vi "New.vi"(4 "Plugin":refnum<class "Plugin.lvclass">, 5 "FIFO Options":T1, 6 "Logging Interface":refnum<class "Logging Interface.lvclass">, 7 "thread ID":u8, 8 "error in (no error)":errorcluster, 10 "Thread Configuration":refnum<class "Thread Configuration.lvclass">, 11 "Plugin Thread type":refnum<class "Plugin Thread.lvclass">) -> (0 "error out":errorcluster, 2 "Plugin Thread Interface":refnum<class "Plugin Interface.lvclass">, 3 "Plugin Thread out":refnum<class "Plugin Thread.lvclass">)   [LabVIEW 2019, in "DSF Core.lvlib" / "Plugin Thread.lvclass"]
uses:
  Thread/Plugin/Plugin Thread.lvclass
  C:/Dev/GitHub/niveristand-data-sharing-framework-custom-device/Core/Classes/Thread/Thread.lvclass
  Interface/Plugin/Plugin Interface.lvclass
  C:/Dev/GitHub/niveristand-data-sharing-framework-custom-device/Core/Classes/Interface/Interface.lvclass
  Configuration/Core/Thread/Thread Configuration.lvclass
  Interface/Logging/Logging Interface.lvclass
  Plugin/Plugin.lvclass
  Typedefs/DSF FIFO Options.ctl
  Interface/Interface.lvclass/Interface.ctl
  Thread/Thread.lvclass/Thread.ctl
  Plugin/Plugin.lvclass/Plugin.ctl
  Timing/Timing.lvclass/Timing.ctl
  Thread/Thread Settings.ctl
  Thread/Plugin/Plugin Thread.lvclass/Plugin Thread.ctl
  Interface/New Interface.vi
  Interface/Create RT FIFO.vi
  Thread/Thread.lvclass
  Timing/Timing.lvclass
  Framework/Framework.lvclass
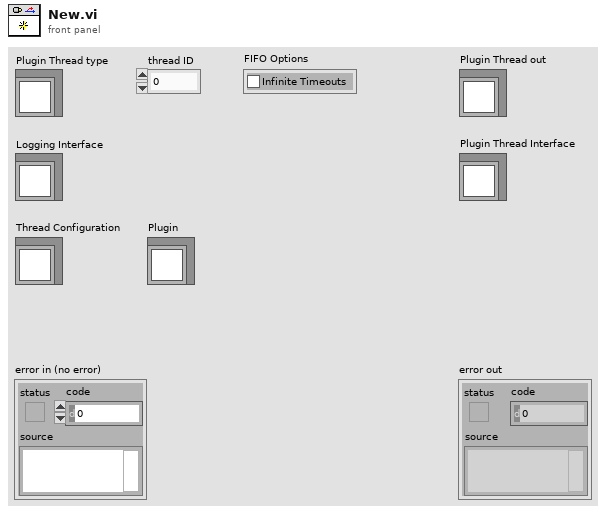
[diagram p1: front panel]
types:
  T1 = typedef "DSF Core.lvlib/Framework.lvclass/DSF FIFO Options.ctl" = cluster{"Infinite Timeouts":bool}
  T2 = typedef "DSF Core.lvlib/Thread.lvclass/Thread Settings.ctl" = cluster{"Priority":u16, "Processor":i32}
  T3 = typedef "DSF Core.lvlib/Thread Configuration.lvclass/Core Thread Configuration.ctl" = cluster{"processor":i32, "priority offset":i16}
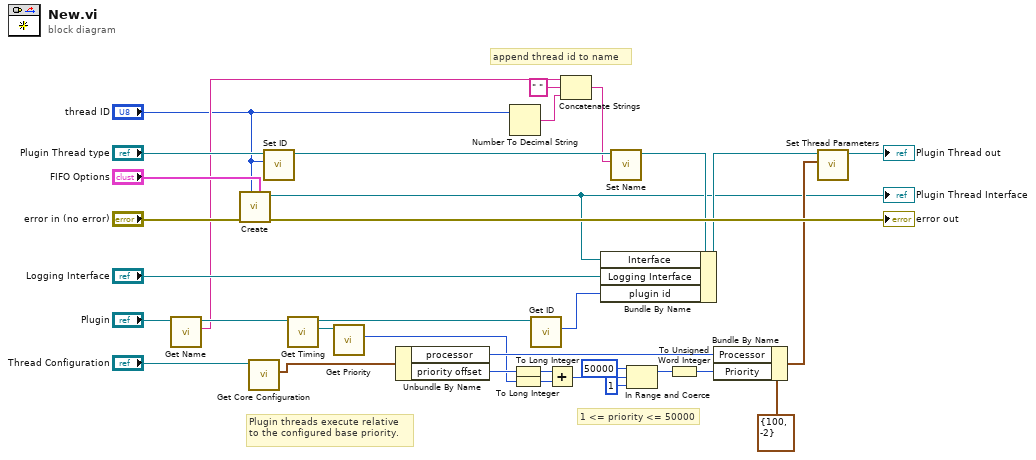
[diagram p0: block diagram]
diagram:
  # "1 <= priority <= 50000"
  # "append thread id to name"
  # "Plugin threads execute relative to the configured base priority."
  n1 = call "Get Name.vi"("Plugin in"="Plugin") -> ("name"=w4:string, "Plugin out"=w12:refnum<class "Plugin.lvclass">)  [unwired: 9 in]
  n2 = call "Create.vi"("fifo options"="FIFO Options", "id (0)"="thread ID", "error in (no error)"="error in (no error)") -> ("error out"=→"error out":errorcluster, "Plugin Interface"=w6:refnum<class "Plugin Interface.lvclass">)  [unwired: 7 in]
  "Plugin Thread Interface" <- w6
  n3 = call "Get Core Configuration.vi"("Thread Configuration in"="Thread Configuration") -> ("core"=w1:T3)  [unwired: 8 in, 2 out]
  n4 = call "Set ID.vi"("ID"="thread ID", "Thread in"="Plugin Thread type") -> ("Thread out"=w9:refnum<class "Plugin Thread.lvclass">)  [unwired: 9 in]
  n5 = call "Get Timing.vi"("Plugin in"=w12) -> ("Timing"=w17:refnum<class "Timing.lvclass">, "Plugin out"=w15:refnum<class "Plugin.lvclass">)  [unwired: 9 in]
  n6 = call "Get Priority.vi"("Timing in"=w17) -> ("Priority"=w16:u16)  [unwired: 9 in, 1 out]
  n7 = Unbundle By Name(w1) -> ("processor"=w24:i32, "priority offset"=w25:i16)
  n8 = Number To Decimal String(number="thread ID") -> (decimal integer string=w20:string)  [unwired: 1 in]
  n9 = To Long Integer(number=w25) -> (32bit integer=w32:i32)
  n10 = To Long Integer(number=w16) -> (32bit integer=w31:i32)
  n11 = call "Get ID.vi"("Plugin in"=w15) -> ("id"=w14:i32)  [unwired: 9 in, 1 out]
  n12 = Add(x=w32, y=w31) -> (x+y=w30:i32)
  n13 = Concatenate Strings(w4, " ", w20) -> (w8:string)
  n14 = call "Set Name.vi"("name"=w8, "Thread in"=w9) -> ("Thread out"=w21:refnum<class "Plugin Thread.lvclass">)  [unwired: 9 in]
  n15 = Bundle By Name(cluster=w21, "Interface"=w6, "Logging Interface"="Logging Interface", "plugin id"=w14) -> (w23:refnum<class "Plugin Thread.lvclass">)
  n16 = In Range and Coerce(upper limit=50000, x=w30, lower limit=1) -> (coerced(x)=w26:i32)  [unwired: 1 out]
  n17 = To Unsigned Word Integer(number=w26) -> (unsigned 16bit integer=w29:u16)
  n18 = Bundle By Name(cluster=T2 {"Priority"=100, "Processor"=-2} ("thread settings"), "Processor"=w24, "Priority"=w29) -> (w22:T2)
  n19 = call "Set Thread Parameters.vi"("thread settings"=w22, "Thread in"=w23) -> ("Thread out"=→"Plugin Thread out":refnum<class "Plugin Thread.lvclass">)  [unwired: 9 in]
